vi "CalculateBand.vi"(0 "Waveform":waveform(sgl), 5 "Feature":T8, 7 "Speed [RPM]":dbl, 11 "error in (no error)":errorcluster, 12 "Calculation State in":T1={"Spectrum Init"=FALSE, "Power Spectrum"={"f0"=0.0, "df"=0.0, "magnitude"=[]}, "spectrum info"={"channel name"="", "description"="", "x-axis units"=0, "spectral info"={"spectrum type"=enum."Power [Magnitude^2]", "linear/dB"=enum."linear", "window"=0, "window size"=0, "FFT size"=0}, "engineering units"=0, "custom label"="", "dB reference [EU]"=0.0, "peak units"=enum."rms", "weighting filter"=0, "spectral density?"=FALSE, "unit label"="", "spectrum skewed?"=FALSE, "complimentary spectrum units"=enum."none"}} {"spectrum info"."x-axis units" items=["Time (s)"=0, "Frequency-CB (Hz)"=1, "Frequency-CPB (Hz)"=1248, "Frequency-Arbitrary (Hz)"=2357, "Quefrency (s)"=2, "Revolutions (rev)"=3, "Order"=4, "Speed (RPM)"=11, "Speed (rad/s)"=21, "Index"=65535]; "spectrum info"."weighting filter" items=["Linear", "A-weighting", "B-weighting", "C-weighting", "ITU-R 468-4", "Dolby", "CCITT", "C-message", "Wb", "Wc", "Wd", "We", "Wf", "Wh", "Wj", "Wk", "Wm", "AES17 20 kHz lowpass", "AES17 40 kHz lowpass", "AES17 20 kHz highpass", "AES17 40 kHz highpass"]; "spectrum info"."dB reference [EU]" format="%.2f"; "spectrum info"."engineering units" items=["custom..."=0, "V"=1, "A"=21, "C"=30, "pC"=31, "s"=32, "-"=29, "Pa"=2, "N"=20, "g"=3, "m/s^2"=4, "m/s"=5, "m"=6, "mm/s"=12, "mm"=13, "micron/s"=14, "micron"=15, "in/s^2"=7, "in/s"=8, "in"=9, "mil/s"=10, "mil"=11, "rad/s^2"=16, "rad/s"=17, "rad"=18, "deg/s^2"=26, "deg/s"=27, "deg"=28, "RPM"=22, "cycle/s^2"=23, "Hz"=24, "cycle"=25, "strain"=19]; "spectrum info"."spectral info"."window" items=["None "=0, "Hanning"=1, "Hamming"=2, "Blackman-Harris"=3, "Exact Blackman"=4, "Blackman"=5, "Flat Top"=6, "4 Term B-Harris "=7, "7 Term B-Harris"=8, "Low Sidelobe"=9, "Force - Exponential"=10, "Gaussian"=62]}) -> (6 "Band Value":sgl, 14 "Calculation State out":T1={"Spectrum Init"=FALSE, "Power Spectrum"={"f0"=0.0, "df"=0.0, "magnitude"=[]}, "spectrum info"={"channel name"="", "description"="", "x-axis units"=0, "spectral info"={"spectrum type"=enum."Power [Magnitude^2]", "linear/dB"=enum."linear", "window"=0, "window size"=0, "FFT size"=0}, "engineering units"=0, "custom label"="", "dB reference [EU]"=0.0, "peak units"=enum."rms", "weighting filter"=0, "spectral density?"=FALSE, "unit label"="", "spectrum skewed?"=FALSE, "complimentary spectrum units"=enum."none"}} {"spectrum info"."x-axis units" items=["Time (s)"=0, "Frequency-CB (Hz)"=1, "Frequency-CPB (Hz)"=1248, "Frequency-Arbitrary (Hz)"=2357, "Quefrency (s)"=2, "Revolutions (rev)"=3, "Order"=4, "Speed (RPM)"=11, "Speed (rad/s)"=21, "Index"=65535]; "spectrum info"."weighting filter" items=["Linear", "A-weighting", "B-weighting", "C-weighting", "ITU-R 468-4", "Dolby", "CCITT", "C-message", "Wb", "Wc", "Wd", "We", "Wf", "Wh", "Wj", "Wk", "Wm", "AES17 20 kHz lowpass", "AES17 40 kHz lowpass", "AES17 20 kHz highpass", "AES17 40 kHz highpass"]; "spectrum info"."dB reference [EU]" format="%.2f"; "spectrum info"."engineering units" items=["custom..."=0, "V"=1, "A"=21, "C"=30, "pC"=31, "s"=32, "-"=29, "Pa"=2, "N"=20, "g"=3, "m/s^2"=4, "m/s"=5, "m"=6, "mm/s"=12, "mm"=13, "micron/s"=14, "micron"=15, "in/s^2"=7, "in/s"=8, "in"=9, "mil/s"=10, "mil"=11, "rad/s^2"=16, "rad/s"=17, "rad"=18, "deg/s^2"=26, "deg/s"=27, "deg"=28, "RPM"=22, "cycle/s^2"=23, "Hz"=24, "cycle"=25, "strain"=19]; "spectrum info"."spectral info"."window" items=["None "=0, "Hanning"=1, "Hamming"=2, "Blackman-Harris"=3, "Exact Blackman"=4, "Blackman"=5, "Flat Top"=6, "4 Term B-Harris "=7, "7 Term B-Harris"=8, "Low Sidelobe"=9, "Force - Exponential"=10, "Gaussian"=62]}, 15 "error out":errorcluster)   [LabVIEW 2017, in "McsaAnalysisFunctions.lvlib"]
uses:
  <vilib>/addons/InsightCM/Utilities/Analysis/MCSA/McsaAnalysisFunctions.lvlib
  <vilib>/addons/InsightCM/Utilities/Analysis/Shared/controls/Feature.ctl
  <vilib>/addons/InsightCM/Utilities/Analysis/Shared/controls/AmplitudeScale.ctl
  <vilib>/addons/InsightCM/Utilities/Analysis/MCSA/controls/PowerSpectrumCalculationCache.ctl
  <vilib>/addons/_NISVFA/_Shared subVIs/Controls/svc_Spectrum Info.ctl
  <vilib>/addons/_NISVFA/_Shared subVIs/Controls/svc_X-Axis Units.ctl
  <vilib>/addons/_NISVFA/_Shared subVIs/Controls/svc_Spectrum Type.ctl
  <vilib>/addons/_NISVFA/_Shared subVIs/Controls/svc_Engineering Units Text Ring.ctl
  <vilib>/addons/_NISVFA/_Shared subVIs/Controls/svc_Weighting Filter Text Ring.ctl
  <vilib>/addons/_NISVFA/_Shared subVIs/Controls/svc_Complimentary Spectrum Units.ctl
  <vilib>/addons/InsightCM/Utilities/Analysis/Shared/controls/BandConfig.ctl
  <vilib>/addons/InsightCM/Utilities/Analysis/Shared/controls/BandDomain.ctl
  <vilib>/addons/InsightCM/Utilities/Analysis/Shared/controls/BandCalculation.ctl
  <vilib>/addons/InsightCM/Utilities/Analysis/Vibration/subVIs/Band Magnitude - Total (Frequency).vi
  <vilib>/addons/InsightCM/Utilities/Analysis/Vibration/subVIs/Band Magnitude - Peak (Frequency).vi
  <vilib>/addons/InsightCM/Utilities/Analysis/Vibration/subVIs/Band Magnitude - Total (CPM).vi
  <vilib>/addons/InsightCM/Utilities/Analysis/Vibration/subVIs/Band Magnitude - Peak (CPM).vi
  <vilib>/addons/InsightCM/Utilities/Analysis/Vibration/subVIs/Band Magnitude - Total (Orders).vi
  <vilib>/addons/InsightCM/Utilities/Analysis/Vibration/subVIs/Band Magnitude - Peak (Orders).vi
  <vilib>/addons/InsightCM/Utilities/Analysis/Vibration/VibrationAnalysisFunctions.lvlib
  <vilib>/addons/InsightCM/Utilities/Analysis/Shared/AnalysisHelper.lvlib
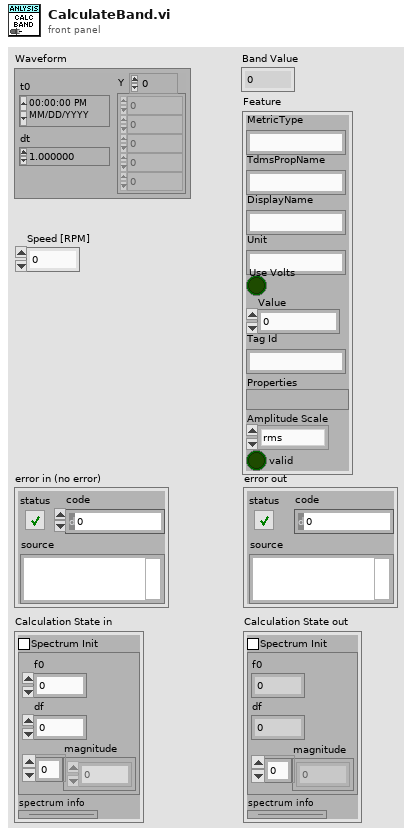
[diagram p1: front panel]
types:
  T1 = typedef "McsaAnalysisFunctions.lvlib/PowerSpectrumCalculationCache.ctl" = cluster{"Spectrum Init":bool, "Power Spectrum":cluster{"f0":dbl, "df":dbl, "magnitude":dbl[]}, "spectrum info":T2}
  T2 = typedef "svc_Spectrum Info.ctl" = cluster{"channel name":string, "description":string, "x-axis units":T3, "spectral info":cluster{"spectrum type":T4, "linear/dB":enum16{"linear", "dB"}, "window":u16, "window size":i32, "FFT size":i32}, "engineering units":T5, "custom label":string, "dB reference [EU]":dbl, "peak units":enum16{"rms", "peak", "peak-peak"}, "weighting filter":T6, "spectral density?":bool, "unit label":string, "spectrum skewed?":bool, "complimentary spectrum units":T7}
  T3 = typedef "svc_X-Axis Units.ctl" = u16
  T4 = typedef "svc_Spectrum Type.ctl" = enum16{"FFT Spectrum [complex]", "Amplitude [Magnitude]", "Power [Magnitude^2]", "Cross Spectrum [complex]", "Frequency Response [Complex]"}
  T5 = typedef "svc_Engineering Units Text Ring.ctl" = u16
  T6 = typedef "svc_Weighting Filter Text Ring.ctl" = u16
  T7 = typedef "svc_Complimentary Spectrum Units.ctl" = enum16{"none", "radians", "degrees", "cycles", "imaginary"}
  T8 = typedef "AnalysisHelper.lvlib/Feature.ctl" = cluster{"MetricType":string, "TdmsPropName":string, "DisplayName":string, "Unit":string, "Use Volts":bool, "Value":dbl, "Tag Id":string, "Properties":variant, "Amplitude Scale":T9, "valid":bool}
  T9 = typedef "AnalysisHelper.lvlib/AmplitudeScale.ctl" = enum16{"rms", "peak", "pk-pk"}
  T10 = typedef "AnalysisHelper.lvlib/BandConfig.ctl" = cluster{"High":dbl, "Low":dbl, "Domain":T11, "Calculation":T12}
  T11 = typedef "AnalysisHelper.lvlib/BandDomain.ctl" = enum16{"Frequency", "CPM", "Orders"}
  T12 = typedef "AnalysisHelper.lvlib/BandCalculation.ctl" = enum16{"Total", "Max", "Phase"}
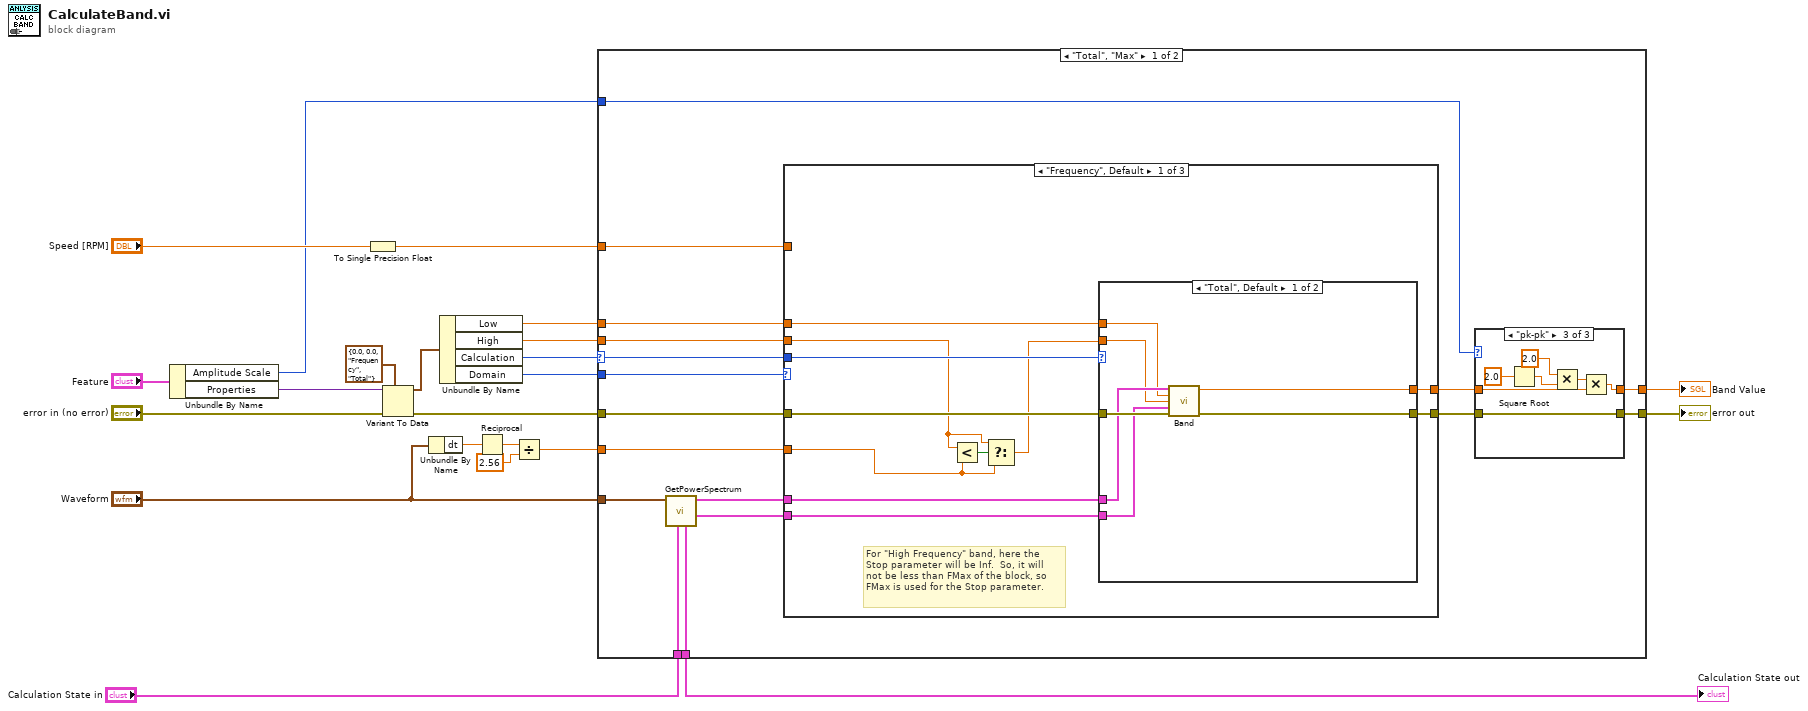
[diagram p0: block diagram]
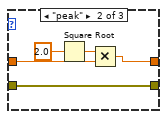
[diagram p3: hidden frame]
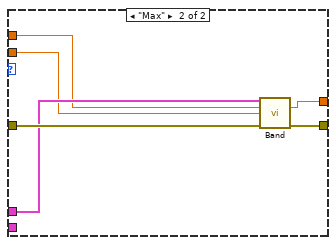
[diagram p4: hidden frame]
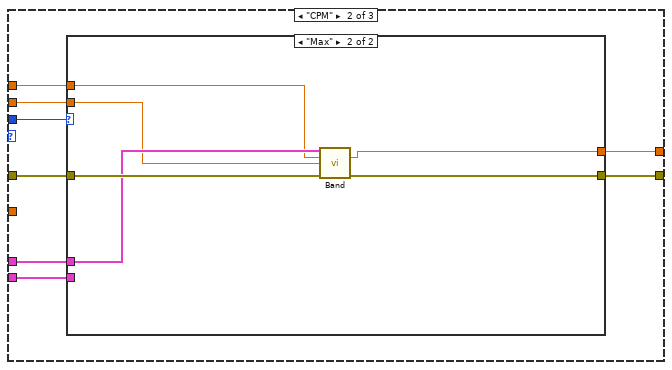
[diagram p5: hidden frame]
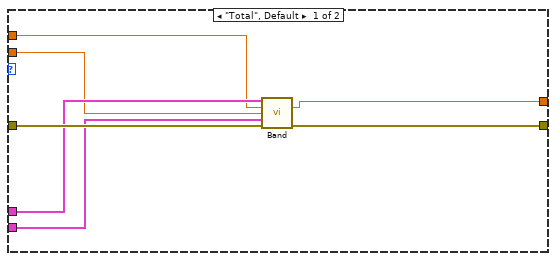
[diagram p6: hidden frame]
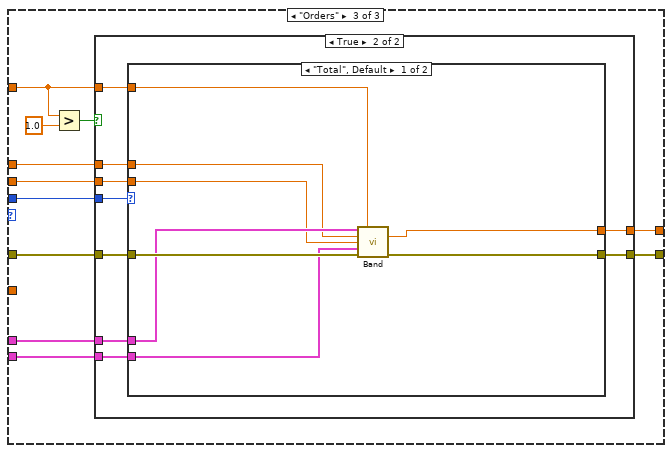
[diagram p7: hidden frame]
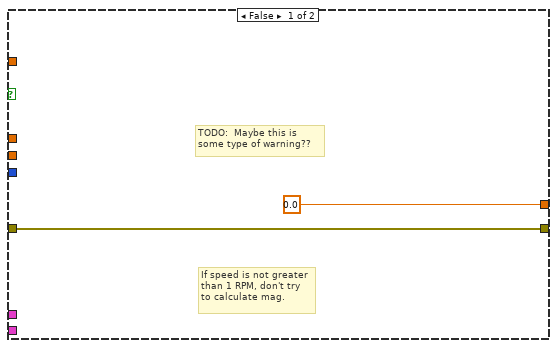
[diagram p8: hidden frame]
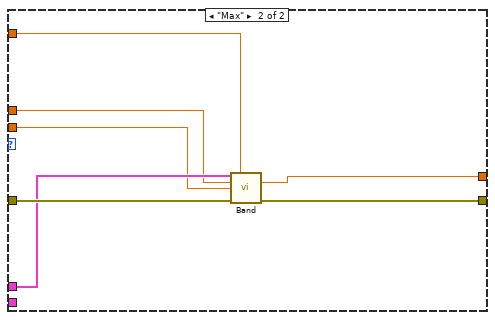
[diagram p9: hidden frame]
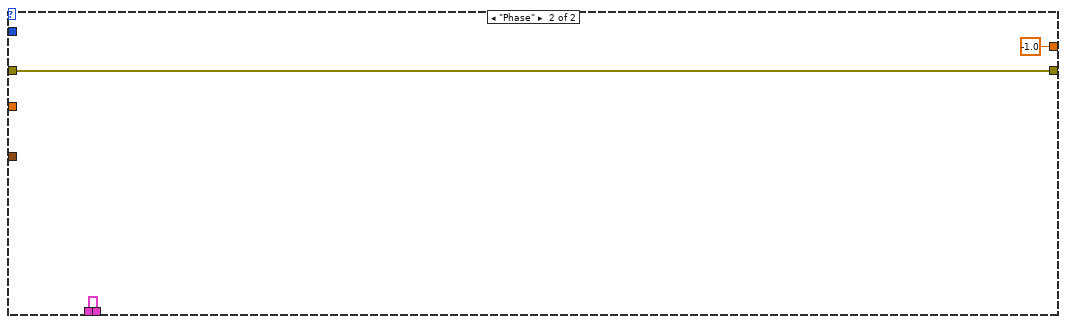
[diagram p10: hidden frame]
diagram:
  n1 = Unbundle By Name("Feature") -> ("Amplitude Scale"=w5:T9, "Properties"=w6:variant)
  n2 = To Single Precision Float(number="Speed [RPM]") -> (single precision float=w1:sgl)
  n3 = Variant To Data(error in="error in (no error)", type=T10 {"High"=0.0, "Low"=0.0, "Domain"=enum."Frequency", "Calculation"=enum."Total"} ("SpectralBand"), Variant=w6) -> (data=w12:T10, error out=w14:errorcluster)
  n4 = Unbundle By Name("Waveform") -> ("dt"=w16:dbl)
  n5 = Unbundle By Name(w12) -> ("Low"=w11:dbl, "High"=w10:dbl, "Calculation"=w9:T12, "Domain"=w8:T11)
  n6 = Reciprocal(x=w16) -> (1/x=w17:dbl)
  n7 = Divide(x=w17, y=2.56) -> (x/y=w18:dbl)
  n8 = case shown="\"Total\", \"Max\"" w9 {
    selector: w9 -> [w34 _]
    tunnel: w14 -> [w39 w137]
    tunnel: w8 -> [w38 _]
    tunnel: w1 -> [w37 _]
    tunnel: [w28 -1.0 ("Max Peak in Band [EU rms]")] -> w21
    tunnel: [w32 w137] -> w20
    tunnel: w10 -> [w36 _]
    tunnel: w11 -> [w35 _]
    tunnel: "Waveform" -> [w27 _]
    tunnel: "Calculation State in" -> [w26 w138]
    tunnel: [w25 w138] -> w2
    tunnel: w18 -> [w33 _]
    tunnel: w5 -> [w29 _]
    frame "Total", "Max" {
      n9 = call <vilib>:"GetPowerSpectrum.vi"("Calculation Cache in"=w26, "Waveform"=w27) -> ("spectrum info"=w23:T2, "power spectrum [EU^2 rms]"=w24:cluster{"f0":dbl, "df":dbl, "magnitude":dbl[]}, "Calculation Cache out"=w25:T1)  [unwired: 7 in]
      n10 = case shown="\"Frequency\", Default" w38 {
        tunnel: w39 -> [w64 w85 w109]
        tunnel: [w61 w84 w108] -> w31
        tunnel: w24 -> [w58 w82 w107]
        tunnel: w23 -> [w63 w81 w106]
        tunnel: [w62 w83 w102] -> w30
        tunnel: w37 -> [_ _ w104]
        tunnel: w36 -> [w56 w79 w101]
        tunnel: w35 -> [w60 w80 w100]
        tunnel: w34 -> [w59 w78 w99]
        tunnel: w33 -> [w54 _ _]
        frame "Frequency", Default {
          # "For \"High Frequency\" band, here the\nStop parameter will be Inf.  So, it will\nnot be less than FMax of the block, so\nFMax is used for the Stop parameter."
          n11 = Less?(x=w56, y=w54) -> (x < y?=w57:bool)
          n12 = Select(t=w56, s=w57, f=w54) -> (s? t:f=w55:dbl)
          n13 = case shown="\"Total\", Default" w59 {
            tunnel: w64 -> [w71 w77]
            tunnel: w58 -> [w70 w76]
            tunnel: w63 -> [w69 _]
            tunnel: [w68 w75] -> w62
            tunnel: [w67 w74] -> w61
            tunnel: w60 -> [w66 w73]
            tunnel: w55 -> [w65 w72]
            frame "Total", Default {
              n14 = call-poly <vilib>:"Band.vi"("power spectrum [EU^2 rms]"=w70, "Start"=w66, "Stop"=w65, "spectrum info"=w69, "error in (no error)"=w71) -> ("Total Magnitude [EU rms]"=w68:sgl, "error out"=w67:errorcluster)  [unwired: 9 in]
            }
            frame "Max" {
              n15 = call-poly <vilib>:"Band.vi"("power spectrum [EU^2 rms]"=w76, "Start"=w73, "Stop"=w72, "error in (no error)"=w77) -> ("Max Peak in Band [EU rms]"=w75:sgl, "error out"=w74:errorcluster)  [unwired: 10 in]
            }
          }
        }
        frame "CPM" {
          n16 = case shown="\"Max\"" w78 {
            tunnel: w85 -> [w92 w98]
            tunnel: [w91 w97] -> w84
            tunnel: [w90 w96] -> w83
            tunnel: w82 -> [w89 w95]
            tunnel: w81 -> [w88 _]
            tunnel: w80 -> [w87 w94]
            tunnel: w79 -> [w86 w93]
            frame "Total", Default {
              n17 = call-poly <vilib>:"Band.vi"("power spectrum [EU^2 rms]"=w89, "Start"=w87, "Stop"=w86, "spectrum info"=w88, "error in (no error)"=w92) -> ("total magnitude [EU rms]"=w90:sgl, "error out"=w91:errorcluster)  [unwired: 9 in]
            }
            frame "Max" {
              n18 = call-poly <vilib>:"Band.vi"("power spectrum [EU^2 rms]"=w95, "Start"=w94, "Stop"=w93, "error in (no error)"=w98) -> ("Max Peak In Band [EU rms]"=w96:sgl, "error out"=w97:errorcluster)  [unwired: 10 in]
            }
          }
        }
        frame "Orders" {
          n19 = Greater?(x=w104, y=sgl 1.0) -> (0:w103:bool)
          n20 = case shown="True" w103 {
            tunnel: w109 -> [w111 w120]
            tunnel: [w111 w115] -> w108
            tunnel: w107 -> [_ w119]
            tunnel: w106 -> [_ w118]
            tunnel: w104 -> [_ w117]
            tunnel: [sgl 0.0 ("Power in Band [EU^2 rms]") w116] -> w102
            tunnel: w101 -> [_ w114]
            tunnel: w100 -> [_ w113]
            tunnel: w99 -> [_ w112]
            frame False {
              # "TODO:  Maybe this is\nsome type of warning??"
              # "If speed is not greater\nthan 1 RPM, don't try\nto calculate mag."
            }
            frame True {
              n21 = case shown="\"Total\", Default" w112 {
                tunnel: w120 -> [w128 w135]
                tunnel: w119 -> [w127 w134]
                tunnel: w118 -> [w126 _]
                tunnel: w117 -> [w125 w133]
                tunnel: [w124 w132] -> w116
                tunnel: [w123 w131] -> w115
                tunnel: w114 -> [w122 w130]
                tunnel: w113 -> [w121 w129]
                frame "Total", Default {
                  n22 = call-poly <vilib>:"Band.vi"("power spectrum [EU^2 rms]"=w127, "Speed (RPM)"=w125, "Start"=w121, "Stop"=w122, "spectrum info"=w126, "error in (no error)"=w128) -> ("Total Magnitude [EU rms]"=w124:sgl, "error out"=w123:errorcluster)  [unwired: 8 in]
                }
                frame "Max" {
                  n23 = call-poly <vilib>:"Band.vi"("power spectrum [EU^2 rms]"=w134, "Speed (RPM)"=w133, "Start"=w129, "Stop"=w130, "error in (no error)"=w135) -> ("Max Peak in Band [EU rms]"=w132:sgl, "error out"=w131:errorcluster)  [unwired: 9 in]
                }
              }
            }
          }
        }
      }
      n24 = case shown="\"pk-pk\"" w29 {
        tunnel: [w40 w46 w53] -> w32
        tunnel: w31 -> [w40 w46 w53]
        tunnel: w30 -> [w41 w45 w52]
        tunnel: [w41 w44 w51] -> w28
        frame "rms", Default {
        }
        frame "peak" {
          n25 = Square Root(x=2.0) -> (sqrt(x)=w43:dbl)
          n26 = Multiply(x=w43, y=w45) -> (x*y=w44:dbl)
        }
        frame "pk-pk" {
          n27 = Square Root(x=2.0) -> (sqrt(x)=w48:dbl)
          n28 = Multiply(x=2.0, y=w48) -> (x*y=w49:dbl)
          n29 = Multiply(x=w49, y=w52) -> (x*y=w51:dbl)
        }
      }
    }
    frame "Phase" {
    }
  }
  "error out" <- w20
  "Band Value" <- w21
  "Calculation State out" <- w2
